vi "chooseState.vi"(9 "BallRef":refnum<class "Ball.lvclass">, 10 "OffensiveTeam":refnum<class "Ally.lvclass">, 11 "Utilities in":refnum<class "Utilities.lvclass">) -> (3 "States":enum16{"Halt", "Exit", "GoTo"}(ring))   [LabVIEW 2023]
uses:
  Ball_class/Ball.lvclass
  Ally_class/Ally.lvclass
  Utilities_class/Utilities.lvclass
  Robot_class/Robot.lvclass
  Robot_class/roles.ctl
  Team_class/Team.lvclass/Team.ctl
  Object_class/Object.lvclass/Object.ctl
  Object_class/Read x.vi
  Object_class/Read y.vi
  Team_class/Read RobotRef.vi
  Team_class/Read OffensivePlay.vi
panel:
  in  "Robot":refnum<class "Robot.lvclass">
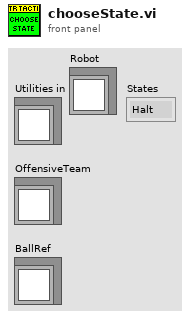
[diagram p1: front panel]
types:
  T1 = typedef "roles.ctl" = enum16{"BallChallengerAttackerVSS", "NormalAttackerVSS", "AttackerAimGoalVSS", "DefenderAreaVSS", "KeeperVSS", "Tabler", "TableFinalizer", "PrepareRollToPassRoller", "PrepareRollToPassReceiver", "SimplePassRoll", "SimplePassRollReceiver", "PenaltyDefense", "PreparePassReceiver 2", "PreparePassReceiver 1", "PassObserver", "Timeout", "Goto", "ZigZag", "None", "BallOutOfField", "DefenderArea", "Duelist", "AttackerStop", "FollowAttacker", "KeeperRole", "KickPenalty", "AttackerAimGoal", "AttackerBlock", "Marker", "Halt", "Shoot", "PassKicker", "PassReceiver", "TestRole", "PenaltyAttacker"}
  T2 = typedef "OffensivePlay.ctl" = enum16{"TableWithStriker", "TableWith2ndStrikerPlay", "PrepareDoublePass", "PrepareRollToPass", "SimplePass", "PreparePass", "PassToStriker", "BallOutOfField", "PassTo2ndStriker", "StopOffensive", "Prepare Penalty Enemy", "EnemyPossessionAtEnemyField", "EnemyPossesionAtOurField", "TestPlay", "PreparePenaltyAlly", "KickPenaltyAlly", "PrepareKickoffAlly", "PrepareKickoffEnemy", "IndirectEnemy", "DirectEnemy", "NormalGame", "DirectKick", "Pass", "Halt", "Timeout", "PassPlay", "PenaltyEnemy"}
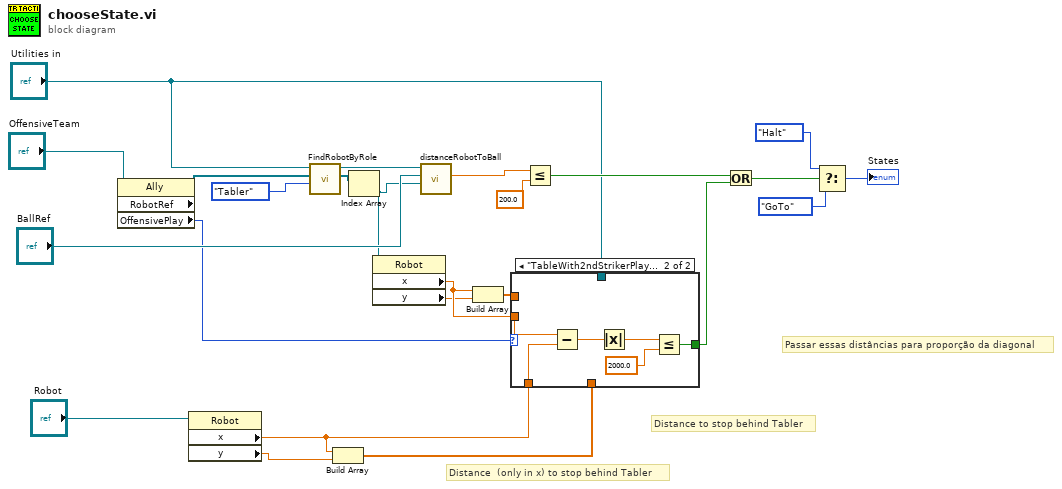
[diagram p0: block diagram]
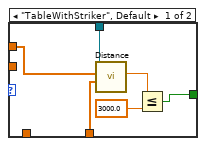
[diagram p2: hidden frame]
diagram:
  # "Passar essas distâncias para proporção da diagonal"
  # "Distance  (only in x) to stop behind Tabler"
  # "Distance to stop behind Tabler"
  n1 = property class="Ally"(reference="OffensiveTeam") -> ("RobotRef"=w15:refnum<class "Robot.lvclass">[], "OffensivePlay"=w12:T2)  [unwired: 1 in, 2 out]
  n2 = property class="Robot"(reference="Robot") -> ("x"=w7:dbl, "y"=w8:dbl)  [unwired: 1 in, 2 out]
  n3 = call "FindRobotByRole.vi"("role"=roles."Tabler", "RobotRef"=w15, "Utilities in"="Utilities in") -> ("Robots"=w18:refnum<class "Robot.lvclass">[], "Utilities out"=w17:refnum<class "Utilities.lvclass">)  [unwired: 6 in, 1 out]
  n4 = Build Array(w7, w8) -> (w6:dbl[])
  n5 = Index Array(array=w18) -> (element=w11:refnum<class "Robot.lvclass">)  [unwired: 1 in]
  n6 = property class="Robot"(reference=w11) -> ("x"=w5:dbl, "y"=w4:dbl)  [unwired: 1 in, 2 out]
  n7 = call "distanceRobotToBall.vi"("Robot"=w11, "Ball"="BallRef", "Utilities in"=w17) -> ("Distance Robot To Ball"=w19:dbl)  [unwired: 6 in, 2 out]
  n8 = Build Array(w5, w4) -> (w3:dbl[])
  n9 = case shown="\"TableWith2ndStrikerPlay\"" w12 {
    tunnel: [w29 w34] -> w2
    tunnel: w5 -> [_ w33]
    tunnel: w7 -> [_ w32]
    tunnel: w3 -> [w27 _]
    tunnel: w6 -> [w28 _]
    tunnel: "Utilities in" -> [w26 _]
    frame "TableWithStriker", Default {
      n10 = call-dynamic "Distance.vi"("P1"=w28, "P2"=w27, "Utilities in"=w26) -> ("Distance"=w30:dbl)  [unwired: 6 in, 2 out]
      n11 = Less Or Equal?(x=w30, y=3000.0) -> (x <= y?=w29:bool)
    }
    frame "TableWith2ndStrikerPlay" {
      n12 = Subtract(x=w33, y=w32) -> (x-y=w36:dbl)
      n13 = Absolute Value(x=w36) -> (abs(x)=w35:dbl)
      n14 = Less Or Equal?(x=w35, y=2000.0) -> (x <= y?=w34:bool)
    }
  }
  n15 = Less Or Equal?(x=w19, y=200.0) -> (x <= y?=w13:bool)
  n16 = Or(x=w13, y=w2) -> (x .or. y?=w1:bool)
  n17 = Select(t=enum16{"Halt", "Exit", "GoTo"}."Halt" ("States"), s=w1, f=enum16{"Halt", "Exit", "GoTo"}."GoTo" ("States")) -> (s? t:f=→"States":enum16{"Halt", "Exit", "GoTo"})
